vi "Open Recordset+.vi"(8 "error in (no error)":errorcluster, 9 "Recordset Parameters":cluster{"CursorType":T1, "LockType":T2}={"CursorType"=1, "LockType"=3} {"LockType" items=["adLockUnspecified"=-1, "adLockReadOnly"=1, "adLockPessimistic"=2, "adLockOptimistic"=3, "adLockBatchOptimistic"=4]; "CursorType" items=["adOpenUnspecified"=-1, "adOpenForwardOnly"=0, "adOpenKeyset"=1, "adOpenDynamic"=2, "adOpenStatic"=3]}, 10 "Source":string, 11 "Connection":refnum<k7>) -> (0 "error out":errorcluster, 3 "Recordset":refnum<k7>)   [LabVIEW 2022 SP3, in "hse-db-ado.lvlib" / "ADO-DB-Driver.lvlib"]
doc: "Open a recordset\n\n____\nHAMPEL SOFTWARE ENGINEERING v1.4.0 (2023-12-19 09:52)"
uses:
  ADO-DB-Driver.lvlib
  _typedefs/CursorType.ctl
  _typedefs/LockType.ctl
panel:
  in  "?":refnum<k7>
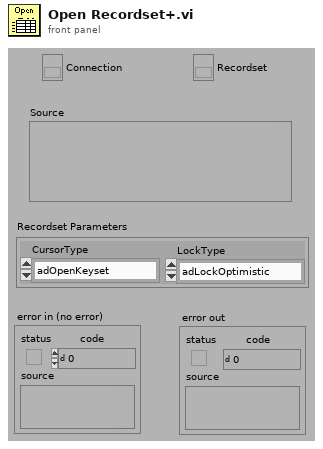
[diagram p1: front panel]
types:
  T1 = typedef "hse-db-ado.lvlib/ADO-DB-Driver.lvlib/CursorType.ctl" = i32
  T2 = typedef "hse-db-ado.lvlib/ADO-DB-Driver.lvlib/LockType.ctl" = i32
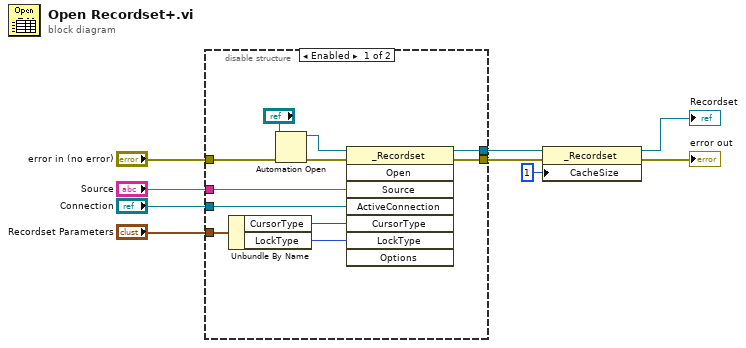
[diagram p0: block diagram]
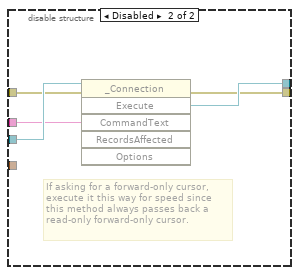
[diagram p2: hidden frame]
diagram:
  n1 = disable-structure shown="Enabled" {
    disable-tunnel: "error in (no error)" -> [w17 w22]
    disable-tunnel: [w16 w24] -> w5
    disable-tunnel: "Connection" -> [w15 w25]
    disable-tunnel: "Recordset Parameters" -> [w14 _]
    disable-tunnel: "Source" -> [w11 w21]
    disable-tunnel: [w10 w23] -> w3
    frame Enabled {
      n2 = Unbundle By Name(w14) -> ("CursorType"=w13:T1, "LockType"=w12:T2)
      n3 = Automation Open(error in (no error)=w17, Automation Refnum="?") -> (Automation Refnum=w20:refnum<k7>, error out=w18:errorcluster)  [unwired: 2 in]
      n4 = invoke class="_Recordset" method="Open"(reference=w20, error in=w18, "Source"=w11, "ActiveConnection"=w15, "CursorType"=w13, "LockType"=w12) -> (reference out=w16:refnum<k7>, error out=w10:errorcluster)  [unwired: 2 in, 6 out]
    }
    frame Disabled {
      # "If asking for a forward-only cursor, \nexecute it this way for speed since \nthis method always passes back a \nread-only forward-only cursor."
      n5 = invoke class="_Connection" method="Execute"(reference=w25, error in=w22, "CommandText"=w21) -> (error out=w23:errorcluster, "Execute"=w24:refnum<k7>)  [unwired: 3 in, 4 out]
    }
  }
  n6 = property class="_Recordset"(reference=w5, error in=w3, "CacheSize"=1) -> (reference out=→"Recordset":refnum<k7>, error out=→"error out":errorcluster)
